vi "StartAcquisition.vi"(8 "error in (no error)":errorcluster, 11 "IVI_Class in":refnum<class "IVI_Class.lvclass">) -> (0 "error out":errorcluster, 3 "IVI_Class out":refnum<class "IVI_Class.lvclass">)   [LabVIEW 2018, in "ScopePlugins.lvlib" / "IVI_Class.lvclass"]
uses:
  IVI_Class.lvclass
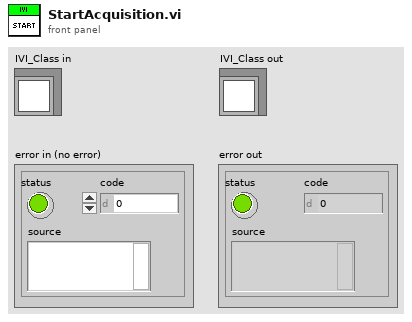
[diagram p1: front panel]
types:
  T1 = typedef "ScopePlugins.lvlib/ScopePluginsBase.lvclass/ChannelSetting(s).ctl" = cluster{"Number of Channels":i32, "Channel(s)":cluster{"Enabled":bool, "Instrument Handle":string, "Channel Name":string, "Maximum Input Frequency":dbl, "Verticle Settings":cluster{"Vertical Range":dbl, "Vertical Offset":dbl, "Probe Attenuation":dbl, "Vertical Coupling":i32}, "Connected":bool, "Input Impedance":dbl, "IO Type Instrument Handle":refnum<k15>}[]}
  T2 = typedef "ScopePlugins.lvlib/ScopePluginsBase.lvclass/HorizontalSettings.ctl" = cluster{"Continuous":bool, "EnableAveraging":bool, "Number Averages":i32, "Measurement Timeout":dbl, "Min Record Length":i32, "Min Sample Rate":dbl, "Enforce Realtime":bool, "Sampling Mode ":enum16{"Real Time", "Equivalent Time", "Segment", "Real Time Peak Detect", "Real Time High Resolution", "Peak Detect Segment", "High Resolution Segment"}, "Interpolation":enum16{"No Interpolation", "sin(x)/x", "linear", "1 Point sin(x)/x", "2 Point sin(x)/x", "4 Point sin(x)/x", "8 Point sin(x)/x", "16 Point sin(x)/x"}, "Type":enum16{"Normal", "PeakDetect", "HighRes", "Envelope", "Average"}, "StartTime":dbl, "Time Per Record":dbl, "Number of Points Minimum":i32, "Measurement Name":string, "Measurement RefreshTime (ms)":u32}
  T3 = cluster{"Enabled":bool, "Instrument Handle":string, "Channel Name":string, "Maximum Input Frequency":dbl, "Verticle Settings":cluster{"Vertical Range":dbl, "Vertical Offset":dbl, "Probe Attenuation":dbl, "Vertical Coupling":i32}, "Connected":bool, "Input Impedance":dbl, "IO Type Instrument Handle":refnum<k15>}[]
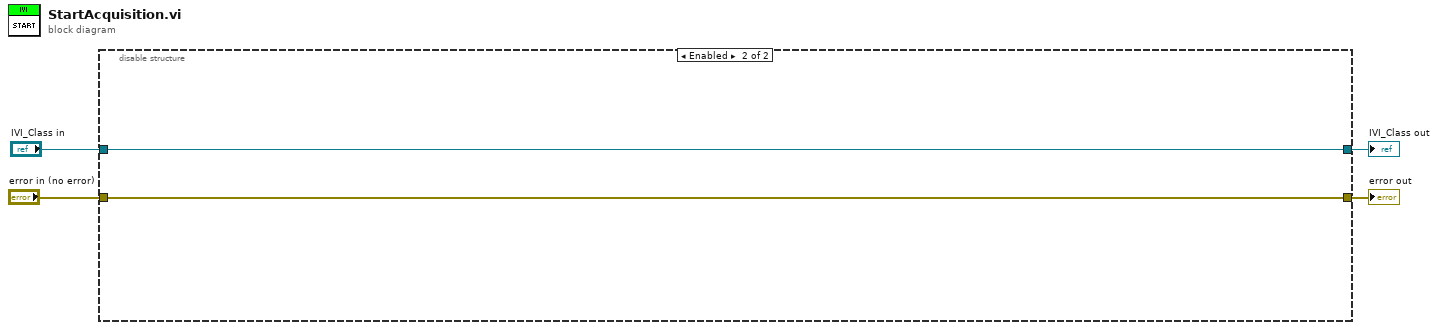
[diagram p0: block diagram]
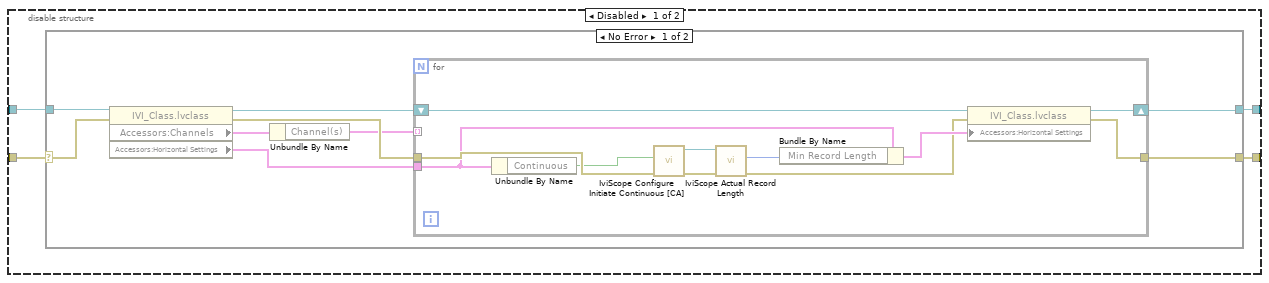
[diagram p2: hidden frame]
diagram:
  n1 = disable-structure shown="Enabled" {
    disable-tunnel: "IVI_Class in" -> [w8 w32]
    disable-tunnel: "error in (no error)" -> [w7 w31]
    disable-tunnel: [w6 w32] -> w2
    disable-tunnel: [w5 w31] -> w1
    frame Disabled {
      n2 = case shown="No Error" w7 {
        selector: w7 -> [w16 w29]
        tunnel: w8 -> [w17 w30]
        tunnel: [w12 w30] -> w6
        tunnel: [w11 w29] -> w5
        frame No Error {
          n3 = property class="IVI_Class.lvclass"(reference=w17, error in=w16) -> (reference out=w15:refnum<class "IVI_Class.lvclass">, error out=w14:errorcluster, "Accessors:Channels"=w10:T1, "Accessors:Horizontal Settings"=w13:T2)
          n4 = Unbundle By Name(w10) -> ("Channel(s)"=w9:T3)
          n5 = for {
            tunnel: w13 -> [w26]
            shift-right: [w25] -> w12
            shift-left: w15 -> [w28]
            tunnel: w14 -> [w27]
            tunnel: [w24] -> w11
            tunnel: w9 -> [_] mode=indexing
            n6 = Unbundle By Name(w26) -> ("Continuous"=w23:bool)
            n7 = call <vilib>:"IviScope Configure Initiate Continuous [CA].vi"("error in (no error)"=w27, "continuous acquisition (Disabled)"=w23) -> ("error out"=w22:errorcluster, "instrument handle out"=w21:refnum<k15>)  [unwired: 8 in]
            n8 = call <vilib>:"IviScope Actual Record Length.vi"("error in (no error)"=w22, "instrument handle"=w21) -> ("error out"=w18:errorcluster, "actual record length"=w20:i32)  [unwired: 8 out]
            n9 = Bundle By Name(cluster=w26, "Min Record Length"=w20) -> (w19:T2)
            n10 = property class="IVI_Class.lvclass"(reference=w28, error in=w18, "Accessors:Horizontal Settings"=w19) -> (reference out=w25:refnum<class "IVI_Class.lvclass">, error out=w24:errorcluster)
          }
        }
        frame Error {
        }
      }
    }
    frame Enabled {
    }
  }
  "error out" <- w1
  "IVI_Class out" <- w2
